vi "Pre-Build Action Debug.vi"(6 "Top Level/Always Included VIs":path[](array[path]), 7 "Main Destination Path":path, 9 "Target Name":string, 10 "Build Specification Name":string, 11 "Project Path":path) -> (0 "error out":errorcluster)   [LabVIEW 2017]
uses:
  Development Tools/Build Automation/Build Automation.lvlib
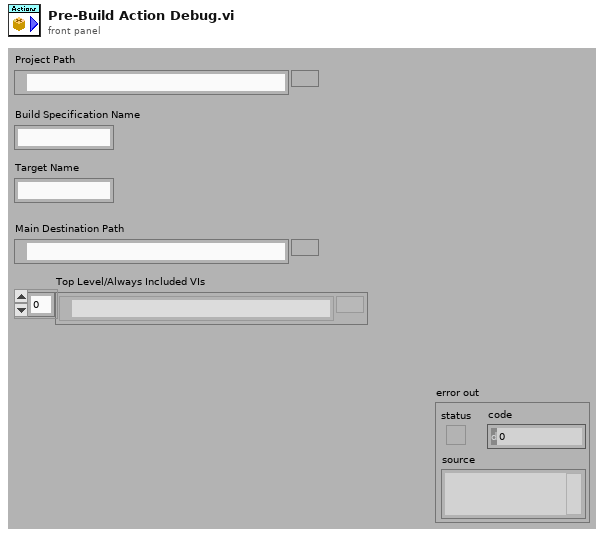
[diagram p1: front panel]
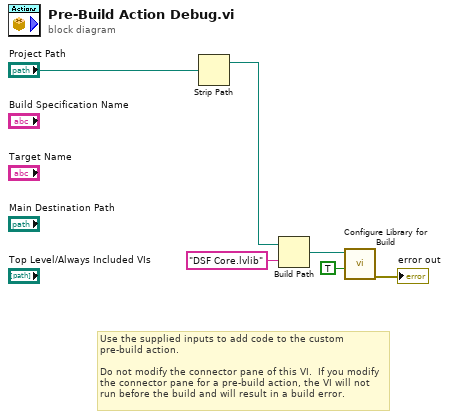
[diagram p0: block diagram]
diagram:
  # "Use the supplied inputs to add code to the custom pre-build action.\n\nDo not modify the connector pane of this VI.  If you modify the connector pane for a pre-build action, the VI will not run before the build and will result in a build error."
  n1 = Strip Path(path="Project Path") -> (stripped path=w1:path)  [unwired: 1 out]
  n2 = Build Path(base path=w1, name or relative path="DSF Core.lvlib" ("library name")) -> (appended path=w3:path)
  n3 = call "Configure Library for Build.vi"("enable debug? (F)"=TRUE, "library path"=w3) -> ("error out"=→"error out":errorcluster)  [unwired: 9 in]
